vi "encode vision points message.vi"(10 "y locations":i16[](array[numeric]) format="%.0x", 11 "x locations":i16[](array[numeric]) format="%.0x") -> (1 "vision points message":u8[](array[numeric]))   [LabVIEW 2009]
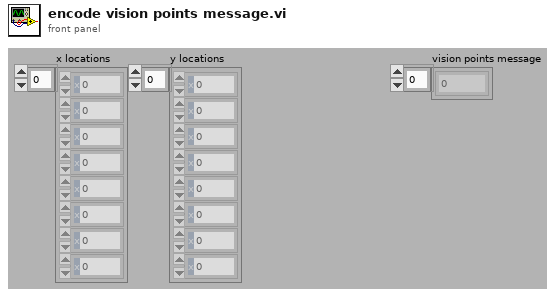
[diagram p1: front panel]
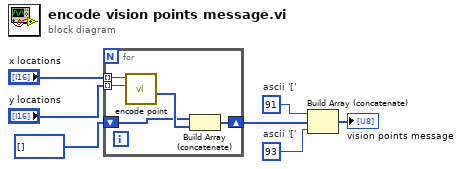
[diagram p0: block diagram]
diagram:
  w3 = u8 93  # ascii '['
  w4 = u8 91  # ascii '['
  n1 = for {
    tunnel: "x locations" -> [w12] mode=indexing
    tunnel: "y locations" -> [w11] mode=indexing
    shift-right: [w9] -> w5
    shift-left: u8[] [] -> [w8]
    n2 = call "encode point.vi"("y"=w11, "x"=w12) -> ("pixel send message"=w10:u8[])  [unwired: 9 in]
    n3 = Build Array (concatenate)(w8, w10) -> (w9:u8[])
  }
  n4 = Build Array (concatenate)(w4, w5, w3) -> (→"vision points message":u8[])
